vi "Acquire data.vi"(8 "error in (no error)":errorcluster, 11 "Gage digitizer actor in":refnum<class "Gage digitizer actor.lvclass">) -> (0 "error out":errorcluster, 3 "Gage digitizer actor out":refnum<class "Gage digitizer actor.lvclass">)   [LabVIEW 2015, in "Gage digitizer actor.lvclass"]
uses:
  Gage digitizer actor.lvclass
  Gage digitizer actor.lvclass/Gage digitizer actor.ctl
  <vilib>/ActorFramework/Actor/Actor.lvclass/Actor.ctl
  <vilib>/ActorFramework/Message Enqueuer/Message Enqueuer.lvclass/Message Enqueuer.ctl
  <vilib>/ActorFramework/Message Enqueuer/Init from Existing Queue.vi
  <vilib>/ActorFramework/Message Enqueuer/Message Enqueuer.lvclass
  Read_Pulse/Control_card.lvclass
  Acquire data request message/Acquired data result msg.lvclass
  <vilib>/ActorFramework/Actor/Actor.lvclass
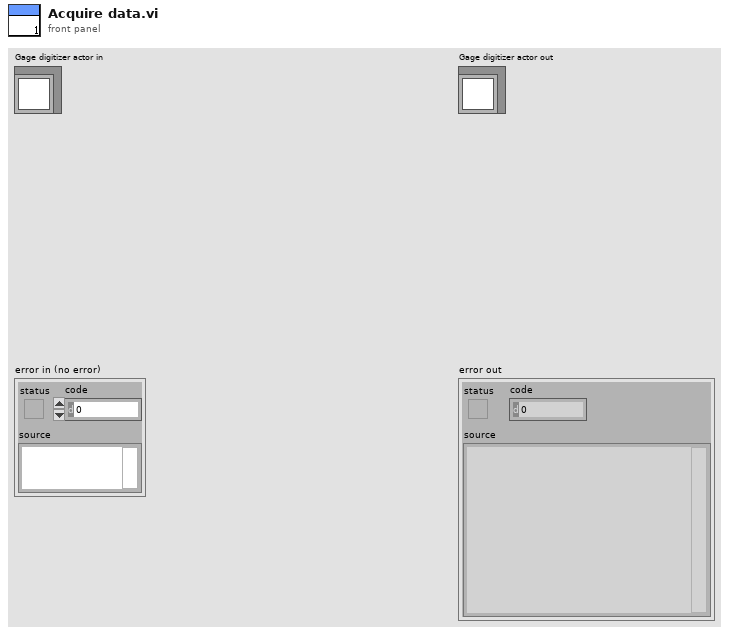
[diagram p1: front panel]
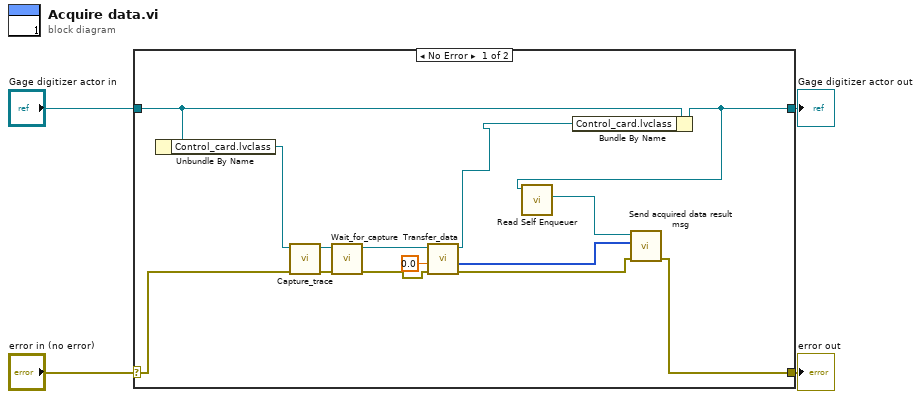
[diagram p0: block diagram]
diagram:
  n1 = case shown="No Error" "error in (no error)" {
    selector: "error in (no error)" -> [w14 w20]
    tunnel: [w7 w20] -> w3
    tunnel: [w5 w19] -> w1
    tunnel: "Gage digitizer actor in" -> [w11 w19]
    frame No Error {
      n2 = Unbundle By Name(w11) -> ("Control_card.lvclass"=w18:refnum<class "Control_card.lvclass">)
      n3 = call-dynamic "Capture_trace.vi"("error in (no error)"=w14, "Initialize_card in"=w18) -> ("error out"=w13:errorcluster, "Initialize_card out"=w17:refnum<class "Control_card.lvclass">)  [unwired: 8 in]
      n4 = call-dynamic "Wait_for_capture.vi"("error in (no error)"=w13, "Initialize_card in"=w17) -> ("error out"=w12:errorcluster, "Initialize_card out"=w16:refnum<class "Control_card.lvclass">)  [unwired: 6 in, 1 out]
      n5 = call-dynamic "Transfer_data.vi"("error in (no error)"=w12, "Start"=0.0, "Initialize_card in"=w16) -> ("error out"=w8:errorcluster, "Data in Volts"=w10:i16[], "Initialize_card out"=w6:refnum<class "Control_card.lvclass">)  [unwired: 6 in]
      n6 = Bundle By Name(cluster=w11, "Control_card.lvclass"=w6) -> (w5:refnum<class "Gage digitizer actor.lvclass">)
      n7 = call <vilib>:"Read Self Enqueuer.vi"("Actor"=w5) -> ("Self Enqueuer"=w9:refnum<class "Message Enqueuer.lvclass">)  [unwired: 10 in]
      n8 = call "Send acquired data result msg.vi"("Message Enqueuer in"=w9, "Data in Volts"=w10, "error in (no error)"=w8) -> ("error out"=w7:errorcluster)  [unwired: 6 in, 1 out]
    }
    frame Error {
    }
  }
  "error out" <- w3
  "Gage digitizer actor out" <- w1
